vi "Image_Processing_Queue.vi"(5 "Data":T4={"Pinch-valve"="Test Sample", "XLP 6000 Pump"="MRJ", "Camera1"="", "Camera2"="", "Img_Capt"=FALSE, "Actuator"=FALSE, "Pump"=FALSE, "Cam 1"=FALSE, "Cam 2"=FALSE, "Empty_Refill"=FALSE, "Crop"=FALSE, "Light intensity"=0, "Exposure Time"=0.0, "Sample Name"="", "Operator"="", "Calibration 1"=path "C:/Users/au540322/Desktop/IHS_Project/images/Debris/Debris_0/Debris_0_2019_06_01-23-32-49-686.PNG", "Calibration 2"=path "C:/Users/au540322/Desktop/IHS_Project/images/Debris/Debris_0/Debris_0_2019_06_01-23-32-49-686.PNG", "Framerate"=1, "Timeout Sample"=1, "Collection date"="", "Sample size threshold"=500, "Empty start"=500, "Command"="", "Station"="", "Species Name"="", "Other Notes"="", "Aperture"=enum."Item 3", "Image Process Queue Size"=100, "Image Save Queue Size"=0, "Overload threshold"=0, "Max Framerate"=0, "Rectangle 1"={"Left"=0, "Top"=0, "Right"=0, "Bottom"=0, "Rotation"=0.0}, "Rectangle 2"={"Left"=0, "Top"=100, "Right"=100, "Bottom"=0, "Rotation"=0.0}, "Detection Region %"=200.0, "Detect 1"=path "C:/Users/au540322/Desktop/IHS_Project/images/Debris/Debris_0/Debris_0_2019_06_01-23-32-49-686.PNG", "Detect 2"=path "C:/Users/au540322/Desktop/IHS_Project/images/Debris/Debris_0/Debris_0_2019_06_01-23-32-49-686.PNG", "Max large object threshold"=500, "Open(T)/Close(F)"=FALSE, "Img_Capt Begin"=FALSE, "Dispense Speed"=0, "Flush Size"=0, "Location"="", "Latitude"="", "Longitude"="", "Determiner"="", "Sex"="", "Camera1_Img"=refnum, "Camera2_Img"=refnum, "Img1_Orig_Disp"=refnum, "Img2_Orig_Disp"=refnum, "Img1_Orig_RGB"=refnum, "Img2_Orig_RGB"=refnum, "Blue_Plane_Extract"=refnum, "Subtracted_Plane"=refnum, "Img1_Binary"=refnum, "Img2_Binary"=refnum, "Crop_Mask"=refnum, "Img1_Save"=refnum, "Img2_Save"=refnum, "Img1_Cali_Full"=refnum, "Img2_Cali_Full"=refnum, "Img1_Cali_Detect"=refnum, "Img2_Cali_Detect"=refnum, "Cam 1 queue"=refnum, "Cam 2 queue"=refnum, "Cam 1 - save queue"=refnum, "Cam 2 - save queue"=refnum, "Overlay_Ring"=0, "SystemVersion"=0, "System Serial"="", "Legacy Cam Attributes"=FALSE, "Camera Orientation 1"="", "Camera Orientation 2"="", "Pixel to mm 1"=0.0, "Pixel to mm 2"=0.0, "CAM1 Model"=enum."a2A5328-15ucBAS", "CAM2 Model"=enum."a2A5328-15ucBAS", "Flush Insect"=FALSE, "Pump Size"=FALSE, "Barcode"="", "Phase3"=FALSE, "Mega F3"="", "Container nr."=0.0, "Flush Error"=TRUE, "Start System"=FALSE, "Size Interval"=0.0, "Mun. of containers"=0.0, "Sorting sys."=FALSE, "Initial size"=0.0} {"SystemVersion" items=["Standard", "XL"]; "Overlay_Ring" items=["Session Data", "Extended Setup", "Buffer", "Camera", "Dispenser", "Stats", "Connections"]; "Flush Size" min=1; "Dispense Speed" min=1; "Rectangle 2"."Rotation" format="%.2f"; "Rectangle 2"."Left" scale=0.0..1024.0; "Rectangle 2"."Right" scale=0.0..1024.0; "Rectangle 1"."Rotation" format="%.2f"; "Rectangle 1"."Left" scale=0.0..1024.0; "Rectangle 1"."Right" scale=0.0..1024.0; "Max Framerate" min=1; "Overload threshold" min=1; "Image Save Queue Size" min=1; "Image Process Queue Size" min=1; "Empty start" min=1; "Sample size threshold" min=1; "Framerate" min=1; "Light intensity" scale=0.0..100.0}) -> (10 "Status":T1, 11 "Detection error":errorcluster, 12 "Process queue":T2, 13 "Last Image?":bool, 14 "Object1":T3, 15 "Object2":T3, 16 "Image 1":T3, 17 "Image 2":T3, 18 "Binary 1":T3, 19 "Binary 2":T3)   [LabVIEW 2024]
doc: "Saves every 6th image in a sub folder in the current directory (specified from Sample Name). When a true is sent to Sample+1 a new subfolder is created with incremental numbering.\nExample of folders: \n../images/Sample_Name/Sample_Name1\n../images/Sample_Name/Sample_Name2"
uses:
  controls/Data.ctl
  <vilib>/userDefined/High Color/IMAQdx.ctl
  <vilib>/vision/Image Controls.llb/IMAQ Image.ctl
  <extravilib>/ChannelInstances/Tag-c(bool,bool)/))Channel.ctl
  Camera_ID.ctl
  <extravilib>/ChannelInstances/Tag-c(bool,bool)/Write With Abort.vi
  <extravilib>/ChannelInstances/Tag-c(bool,bool)/Endpoint.vi
  <extravilib>/ChannelInstances/Tag-c(bool,bool).lvlib
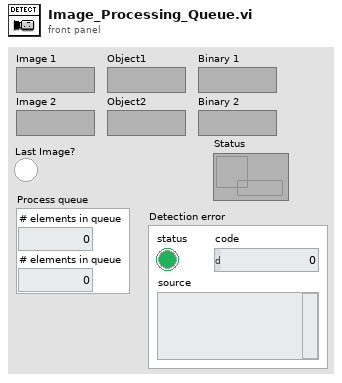
[diagram p1: front panel]
types:
  T1 = typedef "Tag-c(bool,bool).lvlib/))Channel.ctl" = refnum<queue>
  T2 = cluster{"# elements in queue":i32, "# elements in queue":i32}
  T3 = typedef "IMAQ Image.ctl" = refnum<image>
  T4 = typedef "Data.ctl" = cluster{"Pinch-valve":refnum<visa-resource-name>, "XLP 6000 Pump":refnum<visa-resource-name>, "Camera1":T5, "Camera2":T5, "Img_Capt":bool, "Actuator":bool, "Pump":bool, "Cam 1":bool, "Cam 2":bool, "Empty_Refill":bool, "Crop":bool, "Light intensity":i32, "Exposure Time":dbl, "Sample Name":string, "Operator":string, "Calibration 1":path, "Calibration 2":path, "Framerate":i32, "Timeout Sample":i32, "Collection date":string, "Sample size threshold":i32, "Empty start":u32, "Command":string, "Station":string, "Species Name":string, "Other Notes":string, "Aperture":enum32{"Item 0", "Item 1", "Item 2", "Item 3"}, "Image Process Queue Size":i32, "Image Save Queue Size":i32, "Overload threshold":i32, "Max Framerate":i32, "Rectangle 1":T6, "Rectangle 2":T6, "Detection Region %":dbl, "Detect 1":path, "Detect 2":path, "Max large object threshold":i32, "Open(T)/Close(F)":bool, "Img_Capt Begin":bool, "Dispense Speed":i32, "Flush Size":i32, "Location":string, "Latitude":string, "Longitude":string, "Determiner":string, "Sex":string, "Camera1_Img":T3, "Camera2_Img":T3, "Img1_Orig_Disp":T3, "Img2_Orig_Disp":T3, "Img1_Orig_RGB":T3, "Img2_Orig_RGB":T3, "Blue_Plane_Extract":T3, "Subtracted_Plane":T3, "Img1_Binary":T3, "Img2_Binary":T3, "Crop_Mask":T3, "Img1_Save":T3, "Img2_Save":T3, "Img1_Cali_Full":T3, "Img2_Cali_Full":T3, "Img1_Cali_Detect":T3, "Img2_Cali_Detect":T3, "Cam 1 queue":refnum<queue>, "Cam 2 queue":refnum<queue>, "Cam 1 - save queue":refnum<queue>, "Cam 2 - save queue":refnum<queue>, "Overlay_Ring":u16, "SystemVersion":u16, "System Serial":string, "Legacy Cam Attributes":bool, "Camera Orientation 1":string, "Camera Orientation 2":string, "Pixel to mm 1":dbl, "Pixel to mm 2":dbl, "CAM1 Model":enum16{"a2A5328-15ucBAS", "acA1920-155uc"}, "CAM2 Model":enum16{"a2A5328-15ucBAS", "acA1920-155uc"}, "Flush Insect":bool, "Pump Size":bool, "Barcode":string, "Phase3":bool, "Mega F3":refnum<visa-resource-name>, "Container nr.":dbl, "Flush Error":bool, "Start System":bool, "Size Interval":dbl, "Mun. of containers":dbl, "Sorting sys.":bool, "Initial size":dbl}
  T5 = typedef "IMAQdx.ctl" = refnum<k21>
  T6 = typedef "IMAQ Rectangle" = cluster{"Left":i32, "Top":i32, "Right":i32, "Bottom":i32, "Rotation":dbl}
  T7 = typedef "Camera_ID.ctl" = enum16{"Camera 1", "Camera 2"}
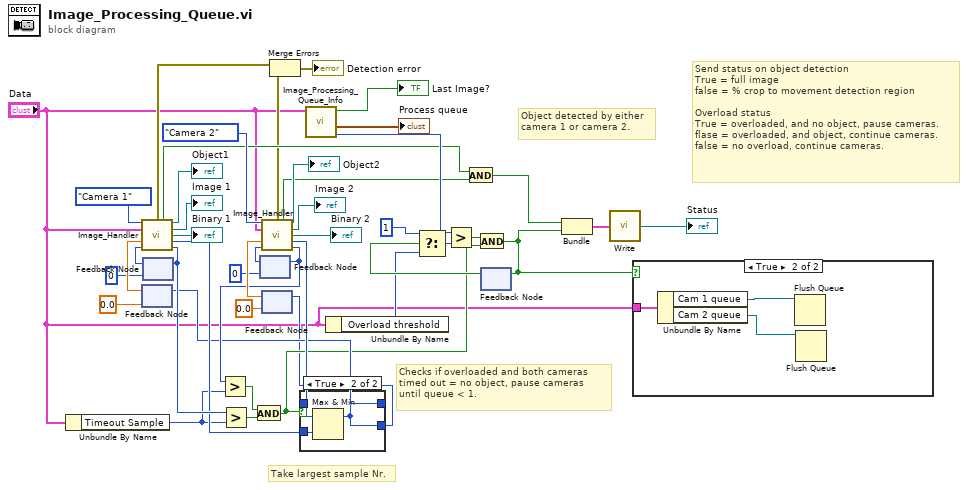
[diagram p0: block diagram]
diagram:
  # "Take largest sample Nr."
  # "Send status on object detection\nTrue = full image\nfalse = % crop to movement detection region\n\nOverload status\nTrue = overloaded, and no object, pause cameras.\nflase = overloaded, and object, continue cameras.\nfalse = no overload, continue cameras."
  # "Object detected by either\ncamera 1 or camera 2."
  # "Checks if overloaded and both cameras \ntimed out = no object, pause cameras \nuntil queue < 1."
  n1 = Unbundle By Name("Data") -> ("Timeout Sample"=w22:i32)
  n2 = feedback #1(0.0 ("Sample nr")) -> (w35:dbl)
  n3 = feedback #2(0 ("Timeout out")) -> (w33:i32)
  n4 = call "Image_Handler.vi"("Camera"=Camera_ID."Camera 1", "Data"="Data", "Prev. sample"=w35, "Timeout in"=w33) -> ("Detection error"=w7:errorcluster, "Object"=w11:bool, "Detected object"=→"Object1":T3, "Image Out"=→"Image 1":T3, "Binary"=→"Binary 1":T3, "Sample nr"=w25:i32, "Timeout out"=w27:i32)  [unwired: 5 in]
  n5 = feedback-in #2(w27) -> ()
  n6 = Greater?(x=w27, y=w22) -> (0:w24:bool)
  n7 = feedback #3(0 ("Timeout out")) -> (w32:i32)
  n8 = feedback #4(0.0 ("Sample nr")) -> (w34:dbl)
  n9 = call "Image_Handler.vi"("Camera"=Camera_ID."Camera 2", "Data"="Data", "Prev. sample"=w34, "Timeout in"=w32) -> ("Detection error"=w8:errorcluster, "Object"=w12:bool, "Detected object"=→"Object2":T3, "Image Out"=→"Image 2":T3, "Binary"=→"Binary 2":T3, "Sample nr"=w26:i32, "Timeout out"=w23:i32)  [unwired: 5 in]
  n10 = Greater?(x=w23, y=w22) -> (0:w21:bool)
  n11 = And(x=w21, y=w24) -> (x .and. y?=w4:bool)
  n12 = feedback-in #3(w23) -> ()
  n13 = Merge Errors(w7, w8) -> (→"Detection error":errorcluster)
  n14 = case shown="True" w4 {
    tunnel: w26 -> [w45 w49]
    tunnel: w25 -> [w46 w48]
    tunnel: [w46 w47] -> w5
    tunnel: [w45 w47] -> w3
    frame False {
    }
    frame True {
      n15 = Max & Min(x=w49, y=w48) -> (max(x,y)=w47:i32)  [unwired: 1 out]
    }
  }
  n16 = feedback-in #1(w5) -> ()
  n17 = feedback-in #4(w3) -> ()
  n18 = call "Image_Processing_Queue_Info.vi"("Data"="Data") -> ("Max Queue Size"=w15:i32, "Queue data"=→"Process queue":T2, "Last Image?"=→"Last Image?":bool)  [unwired: 8 in]
  n19 = Unbundle By Name("Data") -> ("Overload threshold"=w14:i32)
  n20 = And(x=w11, y=w12) -> (x .and. y?=w13:bool)
  n21 = feedback #5() -> (w17:bool)  [unwired: 1 in]
  n22 = Select(t=1 ("y"), s=w17, f=w14) -> (s? t:f=w16:i32)
  n23 = Greater?(x=w15, y=w16) -> (0:w19:bool)
  n24 = And(x=w19, y=w4) -> (x .and. y?=w2:bool)
  n25 = feedback-in #5(w2) -> ()
  n26 = Bundle(w13, w2) -> (w10:cluster{bool, bool})  [unwired: 1 in]
  n27 = call <extravilib>:"Write.vi"("element"=w10) -> ("channel"=→"Status":T1)  [unwired: 1 out]
  n28 = case shown="True" w2 {
    tunnel: "Data" -> [_ w52]
    frame False {
    }
    frame True {
      n29 = Unbundle By Name(w52) -> ("Cam 1 queue"=w51:refnum<queue>, "Cam 2 queue"=w50:refnum<queue>)
      n30 = Flush Queue(queue=w51) -> ()  [unwired: 1 in, 3 out]
      n31 = Flush Queue(queue=w50) -> ()  [unwired: 1 in, 3 out]
    }
  }
